vi "addHeader.vi"(10 "file path (dialog if empty)":path) -> ()   [LabVIEW 2012]
uses:
  <vilib>/Utility/file.llb/Read From Spreadsheet File (string).vi
  <vilib>/Utility/file.llb/Write To Spreadsheet File (string).vi
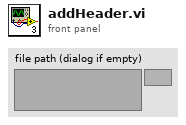
[diagram p1: front panel]
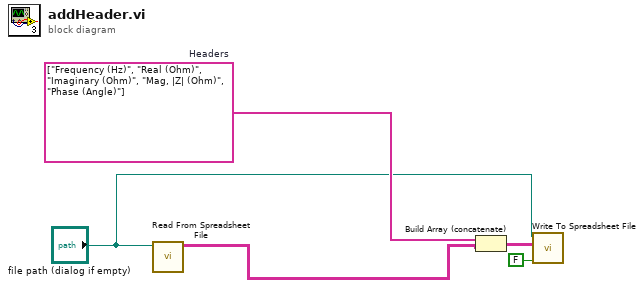
[diagram p0: block diagram]
diagram:
  w4 = string[] ["Frequency (Hz)", "Real (Ohm)", "Imaginary (Ohm)", "Mag, |Z| (Ohm)", "Phase (Angle)"]  # Headers
  n1 = call-poly <vilib>:"Read From Spreadsheet File.vi"("file path (dialog if empty)"="file path (dialog if empty)") -> ("all rows"=w5:string[][])  [unwired: 6 in, 4 out]
  n2 = Build Array (concatenate) "Build Array"(w4, w5) -> (w3:string[][])
  n3 = call-poly <vilib>:"Write To Spreadsheet File.vi"("append to file? (new file:F)"=FALSE, "2D data"=w3, "file path (dialog if empty)"="file path (dialog if empty)") -> ()  [unwired: 5 in, 1 out]
